vi "LaunchBall.vi"(6 "Output":dbl=1.0 format="%#_13g", 8 "error in (no error)":errorcluster, 9 "Timeout (s)":u32, 11 "MotorControlDevRef":T1={"DeviceStatus"={"status"=FALSE, "code"=0, "source"=""}, "Type"=enum."PWM", "PWM"={"Controller"=enum."Controller 1", "PWM Channel"=enum."Invalid", "DeadBand"={"Name"="", "maxPositivePwm"=0, "minPositivePwm"=0, "centerPwm"=0, "maxNegativePwm"=0, "minNegativePwm"=0, "angularRange"=0}}, "CAN"={"Device Number"=0, "Control Mode"=enum."Percent VBus", "Semaphore"=refnum, "Max Vout"=12.0}, "Invert"=FALSE, "TransformRef"=refnum, "InvTransformRef"=refnum}) -> (0 "error out":errorcluster, 3 "MotorControlDevRef 2":T1={"DeviceStatus"={"status"=FALSE, "code"=0, "source"=""}, "Type"=enum."PWM", "PWM"={"Controller"=enum."Controller 1", "PWM Channel"=enum."Invalid", "DeadBand"={"Name"="", "maxPositivePwm"=0, "minPositivePwm"=0, "centerPwm"=0, "maxNegativePwm"=0, "minNegativePwm"=0, "angularRange"=0}}, "CAN"={"Device Number"=0, "Control Mode"=enum."Percent VBus", "Semaphore"=refnum, "Max Vout"=12.0}, "Invert"=FALSE, "TransformRef"=refnum, "InvTransformRef"=refnum})   [LabVIEW 2014]
uses:
  <vilib>/Rock Robotics/WPI/MotorControl/WPI_MotorControlDeviceRef.ctl
  <vilib>/Rock Robotics/SystemInterfaces/Typedef/FPGA_TypedefDigitalModule.ctl
  <vilib>/Rock Robotics/SystemInterfaces/DIO/FPGA_DIOPWMChannel.ctl
  <vilib>/Rock Robotics/WPI/PWM/WPI_PWMDeadband.ctl
  <vilib>/Rock Robotics/WPI/CAN/Jaguar/SubVIs/WPI_CANJaguar_ControlMode.ctl
  <vilib>/Rock Robotics/WPI/PWM/WPI_PWMTransform_ConPane.ctl
  <vilib>/Rock Robotics/WPI/CAN/Jaguar/SubVIs/WPI_CANJaguar_StatusSelect.ctl
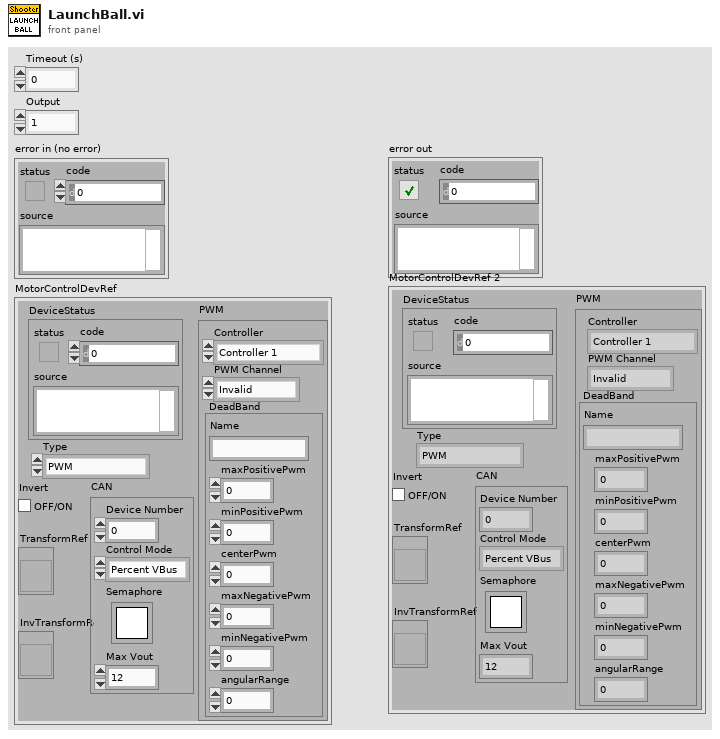
[diagram p1: front panel]
types:
  T1 = typedef "WPI_MotorControlDeviceRef.ctl" = cluster{"DeviceStatus":errorcluster, "Type":enum16{"PWM", "CAN"}, "PWM":cluster{"Controller":T2, "PWM Channel":T3, "DeadBand":T4}, "CAN":cluster{"Device Number":u8, "Control Mode":T5, "Semaphore":T6, "Max Vout":dbl}, "Invert":bool, "TransformRef":T7, "InvTransformRef":T7}
  T2 = typedef "FPGA_TypedefDigitalModule.ctl" = enum16{"Controller 1"}
  T3 = typedef "FPGA_DIOPWMChannel.ctl" = enum8{"PWM 0", "PWM 1", "PWM 2", "PWM 3", "PWM 4", "PWM 5", "PWM 6", "PWM 7", "PWM 8", "PWM 9", "PWM MXP 0", "PWM MXP 1", "PWM MXP 2", "PWM MXP 3", "PWM MXP 4", "PWM MXP 5", "PWM MXP 6", "PWM MXP 7", "PWM MXP 8", "PWM MXP 9", "Invalid"}
  T4 = typedef "WPI_PWMDeadband.ctl" = cluster{"Name":string, "maxPositivePwm":i32, "minPositivePwm":i32, "centerPwm":i32, "maxNegativePwm":i32, "minNegativePwm":i32, "angularRange":u16}
  T5 = typedef "WPI_CANJaguar_ControlMode.ctl" = enum8{"Percent VBus", "Current", "Speed", "Position", "Voltage"}
  T6 = typedef "Semaphore RefNum" = refnum<k1>
  T7 = typedef "WPI_PWMTransform_ConPane.ctl" = refnum<vi>
  T8 = typedef "WPI_CANJaguar_StatusSelect.ctl" = enum16{"Output Percent VBus", "Output Voltage", "Bus Voltage", "Current", "Temperature", "Position", "Speed", "Limit Switches", "Faults", "Fault Counters", "Power Cycle"}
  T9 = typedef "WPI_CANJaguar_Status.ctl" = cluster{"Output Percent VBus":dbl, "Output Voltage":dbl, "Bus Voltage":dbl, "Current":dbl, "Temperature":dbl, "Position":dbl, "Speed":dbl, "Limits":cluster{"Forward Limit":bool, "Reverse Limit":bool, "Forward Soft Limit":bool, "Reverse Soft Limit":bool, "Sticky Forward Limit":bool, "Sticky Reverse Limit":bool, "Sticky Forward Soft Limit":bool, "Sticky Reverse Soft Limit":bool}, "Faults":cluster{"Current Fault":bool, "Temperature Fault":bool, "Bus Voltage Fault":bool, "Gate Driver Fault":bool, "Comm Fault":bool}, "Fault Counters":cluster{"Current Faults":u8, "Temperature Faults":u8, "Bus Voltage Faults":u8, "Gate Driver Faults":u8, "Comm Faults":u8, "CAN Status":u8, "CAN RX Errors":u8, "CAN TX Errors":u8}, "Power Cycle":bool}
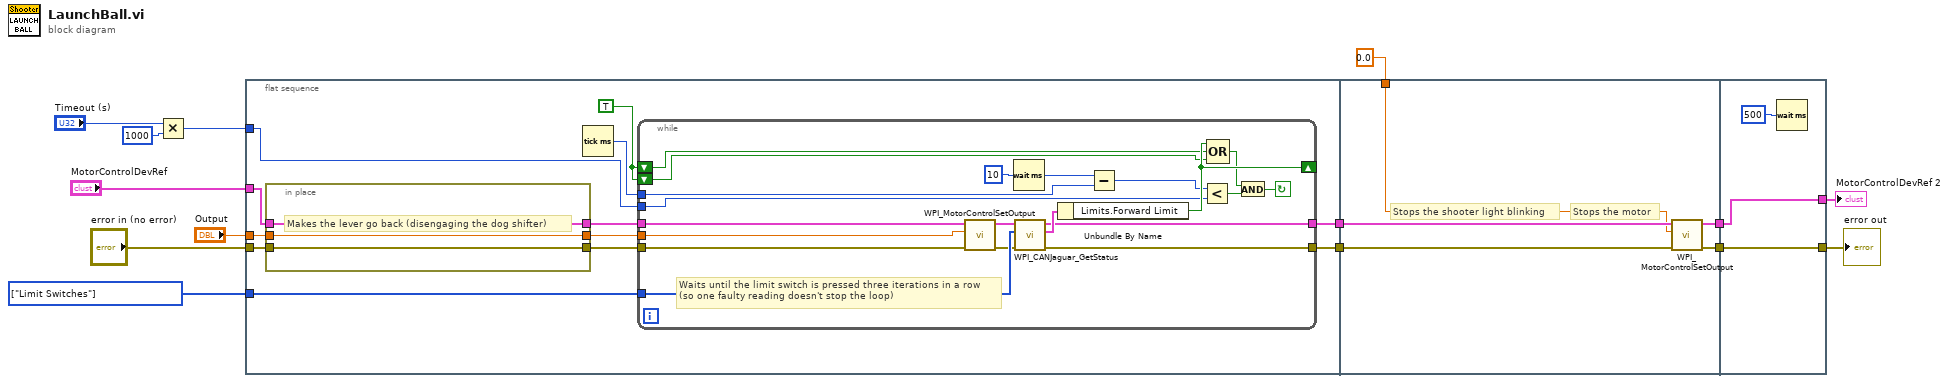
[diagram p0: block diagram]
diagram:
  w11 = T8[] [enum."Limit Switches"] items=["Output Percent VBus", "Output Voltage", "Bus Voltage", "Current", "Temperature", "Position", "Speed", "Limit Switches", "Faults", "Fault Counters", "Power Cycle"] ("Status Select")
  n1 = Multiply(x="Timeout (s)", y=u32 1000) -> (x*y=w4:u32)
  n2 = flat-sequence {
    tunnel: [w25] -> w14
    tunnel: [w26] -> w13
    tunnel: w11 -> [w24]
    tunnel: "Output" -> [w23]
    tunnel: w4 -> [w19]
    tunnel: "error in (no error)" -> [w22]
    tunnel: "MotorControlDevRef" -> [w15]
    tunnel: [w54] -> w10
    tunnel: [w53] -> w9
    tunnel: w13 -> [w51]
    tunnel: w14 -> [w52]
    tunnel: 0.0 ("Output") -> [w50]
    tunnel: w10 -> [w55]
    tunnel: w9 -> [w56]
    tunnel: [w56] -> w7
    tunnel: [w55] -> w1
    frame #0 {
      w21 = TRUE
      n3 = in-place {
        in-place-border: w23 -> [w47]
        in-place-border: w15 -> [w48]
        in-place-border: w22 -> [w49]
        in-place-border: [w49] -> w18
        in-place-border: [w48] -> w17
        in-place-border: [w47] -> w16
        # "Makes the lever go back (disengaging the dog shifter)"
      }
      n4 = Tick Count (ms)() -> (millisecond timer value=w20:u32)
      n5 = while {
        tunnel: w24 -> [w44]
        tunnel: [w43] -> w26
        shift-right: [w42] -> _
        shift-left: w21 -> [w41]
        shift-left: w21 -> [w40]
        tunnel: [w45] -> w25
        tunnel: w20 -> [w35]
        tunnel: w19 -> [w32]
        tunnel: w18 -> [w30]
        tunnel: w17 -> [w29]
        tunnel: w16 -> [w28]
        stop <- w34 continue-if-true
        # "Waits until the limit switch is pressed three iterations in a row\n(so one faulty reading doesn't stop the loop)"
        n6 = call <vilib>:"WPI_MotorControlSetOutput.vi"("error in (no error)"=w30, "Output"=w28, "MotorControlDevRef"=w29) -> ("error out"=w31:errorcluster, "MotorControlDevRef"=w27:T1)  [unwired: 6 in, 1 out]
        n7 = Wait (ms)(milliseconds to wait=u32 10) -> (millisecond timer value=w37:u32)
        n8 = call <vilib>:"WPI_CANJaguar_GetStatus.vi"("error in (no error)"=w31, "Status Select"=w44, "CAN Jaguar Ref"=w27) -> ("error out"=w43:errorcluster, "Status"=w46:T9, "CAN Jaguar Ref Out"=w45:T1)  [unwired: 6 in]
        n9 = Unbundle By Name(w46) -> ("Limits.Forward Limit"=w42:bool)
        n10 = Subtract(x=w37, y=w35) -> (x-y=w38:u32)
        n11 = Less?(x=w38, y=w32) -> (x < y?=w33:bool)
        n12 = Compound Arithmetic op=OR(w42, w41, w40) -> (w39:bool)
        n13 = And(x=w39, y=w33) -> (x .and. y?=w34:bool)
      }
    }
    frame #1 {
      # "Stops the motor"
      # "Stops the shooter light blinking"
      n14 = call <vilib>:"WPI_MotorControlSetOutput.vi"("error in (no error)"=w51, "Output"=w50, "MotorControlDevRef"=w52) -> ("error out"=w53:errorcluster, "MotorControlDevRef"=w54:T1)  [unwired: 6 in, 1 out]
    }
    frame #2 {
      n15 = Wait (ms)(milliseconds to wait=u32 500) -> ()  [unwired: 1 out]
    }
  }
  "error out" <- w7
  "MotorControlDevRef 2" <- w1
